vi "SOUR_POW_CORR_COLL_METH_S.vi"(0 "VISA IN":refnum<visa-resource-name>, 1 "Port number":i32, 2 "Method":string, 5 "error in":errorcluster, 7 "Channel":i32) -> (14 "VISA Out":refnum<visa-resource-name>, 19 "error out":errorcluster)   [LabVIEW 2018, in "PNA-X.lvlib"]
doc: "SOURce<cnum>:POWer<port>:CORRection:COLLect:METHod <char> Superseded \nThis command is replaced with SOUR:POW:CORR:COLLect[:ACQuire] which now specifies the \nmethod and the device. \n(Read-Write) Selects the calibration method to be used for the source power cal acquisition. \nParameters \n<cnum> Any existing channel number. If unspecified, value is set to 1 \n<port> Port number to correct for source power. If unspecified, value is set to 1. \n<char> Choose from: \nNONE - No Cal method \nPMETer - Power Meter is used for all readings. (same as \"fast iteration\" box \nnot checked on dialog box) \nPMReceiver - Power meter for the first iteration; then use the reference \nreceiver for remaining readings if necessary (same as \"fast iteration\" box \n1840\n\nchecked on dialog box) \nExamples SOUR:POW:CORR:COLL:METH PMET \nsource1:power2:correction:collect:method pmreceiver \nQuery Syntax SOURce:POWer:CORRection:COLLect:METHod? \nReturn Type Character \nDefault NONE"
uses:
  PNA-X.lvlib
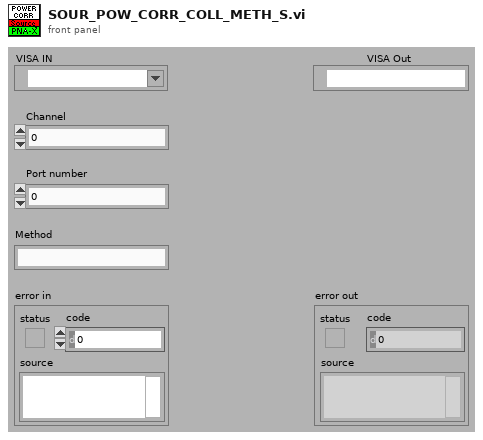
[diagram p1: front panel]
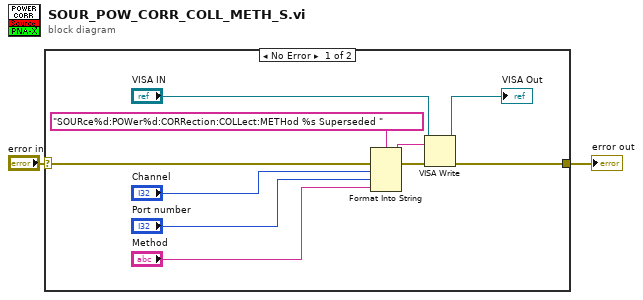
[diagram p0: block diagram]
diagram:
  n1 = case shown="No Error" "error in" {
    selector: "error in" -> [w12 w13]
    tunnel: [w7 w13] -> w1
    frame No Error {
      n2 = Format Into String(format string="SOURce%d:POWer%d:CORRection:COLLect:METHod %s Superseded " ("Cmdline"), error in=w12, "Channel", "Port number", "Method") -> (resulting string=w10:string, error out=w11:errorcluster)  [unwired: 1 in]
      n3 = VISA Write(VISA resource name="VISA IN", write buffer=w10, error in (no error)=w11) -> (VISA resource name out=→"VISA Out":refnum<visa-resource-name>, error out=w7:errorcluster)  [unwired: 1 out]
    }
    frame Error {
    }
  }
  "error out" <- w1
